vi "MultiChannnel_With_Origin_init_Matrix_FileIO.vi"() -> ()   [LabVIEW 2023]
uses:
  <vilib>/Waveform/WDTOps.llb/WDT Index Channel DBL.vi
  <vilib>/Analysis/NI_AALBase.lvlib
  <vilib>/Analysis/baseanly.llb/Mean (DBL).vi
  <vilib>/DAQmx/read.llb/DAQmx Read (Analog 1D Wfm NChan NSamp).vi
  <vilib>/Analysis/Matrix/NI_Matrix.lvlib
  <vilib>/Analysis/baseanly.llb/Real A x B.vi
  <vilib>/DAQmx/configure/timing.llb/DAQmx Timing (Sample Clock).vi
  <vilib>/DAQmx/create/channels.llb/DAQmx Create Channel (AI-Voltage-Basic).vi
  <vilib>/Analysis/Matrix/Numeric/Conversions/Matrix To Array - RM.vi
panel:
  out "attributes 2":variant
  out "attributes":variant
  out "Filename Out":path
  out "Data Writing":bool caption="Saving Data"
  in  "DataWriting SW":bool caption="Enable"
  out "Force Graph":dbl[][](graph)
  out "Force Array (F)   -> Time":dbl[][](array[numeric]) format="%#.3f"
  in  "Convert Matrix":dbl[][](array[numeric])=[[0.01787384, 0.5614992, -0.6825333], [-0.80829626, 0.31005788, 0.3553213], [0.6880116, 0.4358145, 0.7359737]]
  in  "StopAll":bool
  out "How many time get offset":i32
  out "Ch3 Origin":dbl
  out "Ch2 Origin":dbl
  out "Ch1 Origin":dbl
  out "RawCantilever (V)\n (Offset removed     -> Time)":dbl[][](array[numeric]) format="%#.3f"
  out "C 3":dbl[](array[numeric]) format="%#.5g"
  out "C 2":dbl[](array[numeric]) format="%#.5g"
  out "C1":dbl[](array[numeric]) format="%#.5g"
  in  "Get Orogin":bool
  out "Raw AD":waveform(dbl)[](graph)
  in  "samples per channel":i32=500
  in  "sample mode":i32(ring)=10123 items=["Continuous Samples"=10123, "Finite Samples"=10178, "Hardware Timed Single Point"=12522]
  in  "rate":dbl=1000.0 format="%0.2f"
  in  "physical channels":tag="Dev2/ai0:2"
  # "Phy Channel -> Set to 0-2\nRate 1000Hz\nSampleMode  -> Contenious Sampling\nSample per Channel -> 100"
  # "Raw A/D (V)"
  # "C1"
  # "Shear X"
  # "C2"
  # "Shear Y"
  # "Offset (V)"
  # "C3"
  # "Force Z"
  # "No.509 \n[[ 0.01787384, 0.5614992 , -0.6825333 ],\n[-0.80829626, 0.31005788, 0.3553213 ],\n[ 0.6880116 , 0.4358145 , 0.7359737 ]"
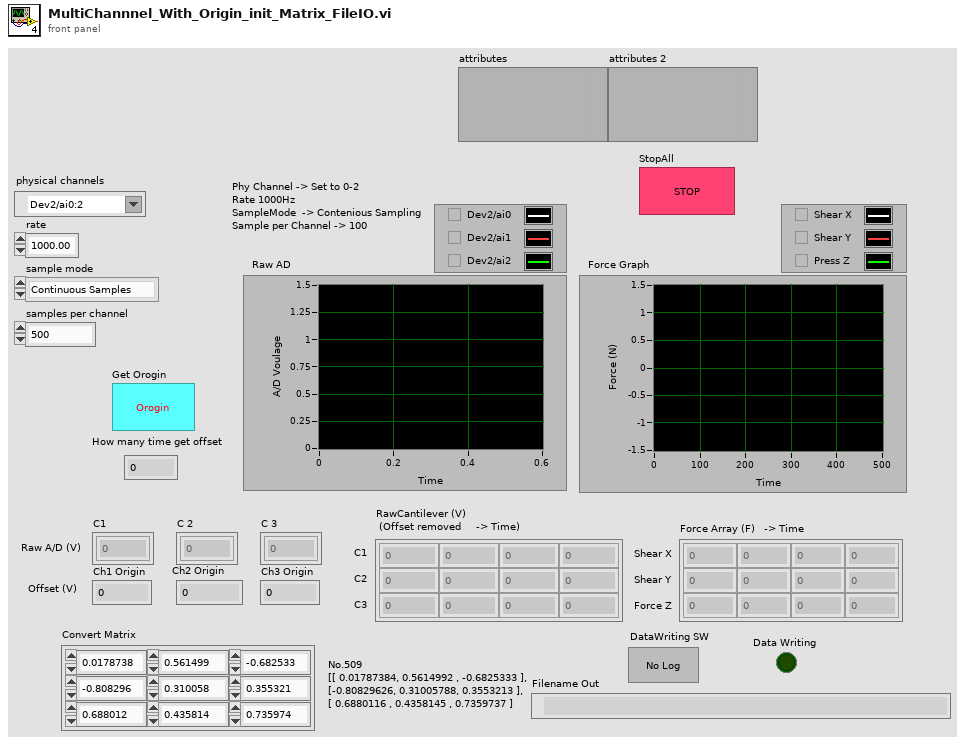
[diagram p1: front panel]
types:
  T1 = typedef "NI_Matrix.lvlib/RealMatrix.ctl" = dbl[][]
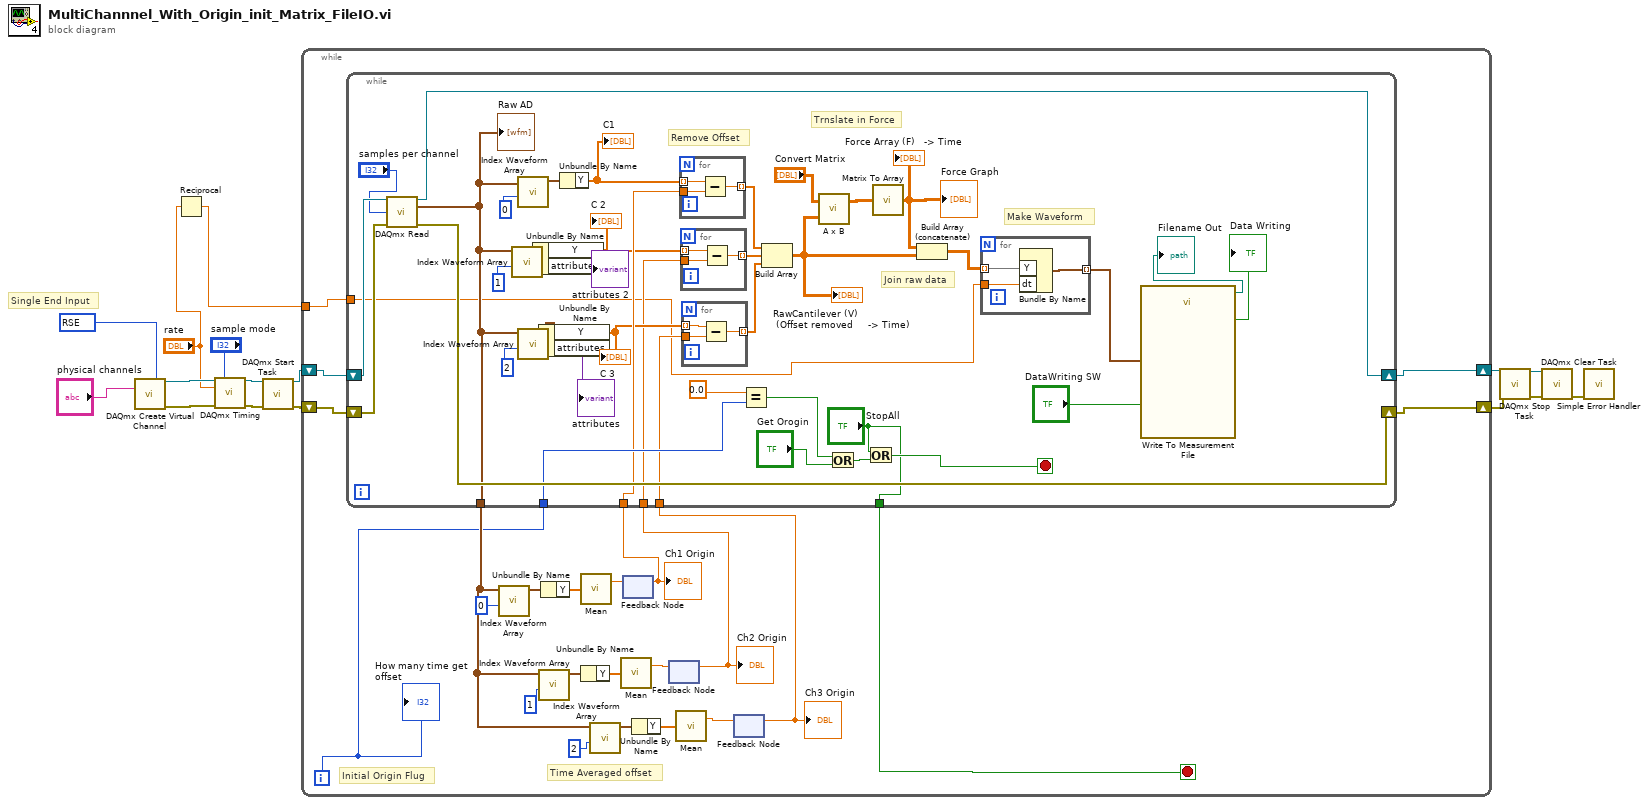
[diagram p0: block diagram]
diagram:
  w3 = 10083 items=["Default"=-1, "RSE"=10083, "NRSE"=10078, "Differential"=10106, "Pseudodifferential"=12529] ("input terminal configuration")
  # "Single End Input"
  n1 = call-poly <vilib>:"DAQmx Create Virtual Channel.vi"("input terminal configuration"=w3, "physical channels"="physical channels") -> ("task out"=w8:refnum<k21>, "error out"=w7:errorcluster)  [unwired: 12 in]
  n2 = Reciprocal(x="rate") -> (1/x=w1:dbl)
  n3 = call-poly <vilib>:"DAQmx Timing.vi"("task/channels in"=w8, "sample mode"="sample mode", "rate"="rate", "error in"=w7) -> ("task out"=w6:refnum<k21>, "error out"=w5:errorcluster)  [unwired: 10 in]
  n4 = call <vilib>:"DAQmx Start Task.vi"("task/channels in"=w6, "error in"=w5) -> ("task out"=w15:refnum<k21>, "error out"=w14:errorcluster)  [unwired: 12 in]
  n5 = while {
    shift-right: [w36] -> w12
    shift-left: w15 -> [w39]
    shift-right: [w37] -> w13
    shift-left: w14 -> [w38]
    tunnel: w1 -> [w17]
    i -> [w27]
    stop <- w28 stop-if-true
    # "Time Averaged offset"
    # "Initial Origin Flug"
    n6 = feedback #1() -> (w23:dbl)  [unwired: 1 in]
    "Ch1 Origin" <- w23
    n7 = feedback #2() -> (w18:dbl)  [unwired: 1 in]
    "Ch2 Origin" <- w18
    n8 = feedback #3() -> (w19:dbl)  [unwired: 1 in]
    "Ch3 Origin" <- w19
    n9 = while {
      shift-right: [w76] -> w36
      shift-left: w39 -> [w79]
      shift-right: [w77] -> w37
      shift-left: w38 -> [w78]
      tunnel: [w50] -> w32
      tunnel: ["StopAll"] -> w28
      tunnel: w27 -> [w65]
      tunnel: w23 -> [w58]
      tunnel: w18 -> [w54]
      tunnel: w19 -> [w53]
      tunnel: w17 -> [w47]
      stop <- w68 stop-if-true
      # "Make Waveform"
      # "Trnslate in Force"
      # "Remove Offset"
      # "Join raw data"
      n10 = call-poly <vilib>:"DAQmx Read.vi"("task/channels in"=w79, "number of samples per channel"="samples per channel", "error in"=w78) -> ("task out"=w76:refnum<k21>, "data"=w50:waveform(dbl)[], "error out"=w77:errorcluster)  [unwired: 10 in]
      "Raw AD" <- w50
      n11 = call-poly <vilib>:"Index Waveform Array.vi"("index"=1, "waveform array"=w50) -> ("waveform"=w71:waveform(dbl))  [unwired: 8 in, 1 out]
      n12 = call-poly <vilib>:"Index Waveform Array.vi"("index"=0, "waveform array"=w50) -> ("waveform"=w73:waveform(dbl))  [unwired: 8 in, 1 out]
      n13 = call-poly <vilib>:"Index Waveform Array.vi"("index"=2, "waveform array"=w50) -> ("waveform"=w69:waveform(dbl))  [unwired: 8 in, 1 out]
      n14 = Unbundle By Name(w71) -> ("Y"=w56:dbl[], "attributes"=→"attributes 2":variant)
      "C 2" <- w56
      n15 = Unbundle By Name(w69) -> ("Y"=w55:dbl[], "attributes"=→"attributes":variant)
      "C 3" <- w55
      n16 = Unbundle By Name(w73) -> ("Y"=w59:dbl[])
      "C1" <- w59
      n17 = for {
        tunnel: w59 -> [w91] mode=indexing
        tunnel: w58 -> [w90]
        tunnel: [w89] -> w57 mode=indexing
        n18 = Subtract(x=w91, y=w90) -> (x-y=w89:dbl)
      }
      n19 = for {
        tunnel: [w88] -> w52 mode=indexing
        tunnel: w56 -> [w87] mode=indexing
        tunnel: w54 -> [w86]
        n20 = Subtract(x=w87, y=w86) -> (x-y=w88:dbl)
      }
      n21 = for {
        tunnel: [w85] -> w51 mode=indexing
        tunnel: w55 -> [w84] mode=indexing
        tunnel: w53 -> [w83]
        n22 = Subtract(x=w84, y=w83) -> (x-y=w85:dbl)
      }
      n23 = Equal?(x=0.0, y=w65) -> (x = y?=w64:bool)
      n24 = Build Array(w57, w52, w51) -> (w45:dbl[][])
      "RawCantilever (V)\n (Offset removed     -> Time)" <- w45
      n25 = call-poly <vilib>:"A x B.vi"("B"=w45, "A"="Convert Matrix") -> ("A x B"=w61:T1)  [unwired: 1 out]
      n26 = Or(x=w64, y="Get Orogin") -> (x .or. y?=w62:bool)
      n27 = Or(x="StopAll", y=w62) -> (x .or. y?=w68:bool)
      n28 = call-poly <vilib>:"Matrix To Array.vi"("Real Matrix"=w61) -> ("Real 2D Array"=w43:dbl[][])
      "Force Array (F)   -> Time" <- w43
      "Force Graph" <- w43
      n29 = Build Array (concatenate)(w43, w45) -> (w44:dbl[][])
      n30 = for {
        tunnel: w44 -> [w80] mode=indexing
        tunnel: [w82] -> w46 mode=indexing
        tunnel: w47 -> [w81]
        n31 = Bundle By Name("Y"=w80, "dt"=w81) -> (w82:waveform(dbl))  [unwired: 1 in]
      }
      n32 = call "Write To Measurement File"("Signals"=w46, "Enable"="DataWriting SW") -> ("Filename Out"=→"Filename Out":path, "Saving Data"=→"Data Writing":bool)  [unwired: 15 in, 1 out]
    }
    n33 = call-poly <vilib>:"Index Waveform Array.vi"("index"=0, "waveform array"=w32) -> ("waveform"=w35:waveform(dbl))  [unwired: 8 in, 1 out]
    n34 = call-poly <vilib>:"Index Waveform Array.vi"("index"=1, "waveform array"=w32) -> ("waveform"=w34:waveform(dbl))  [unwired: 8 in, 1 out]
    n35 = Unbundle By Name(w35) -> ("Y"=w26:dbl[])
    n36 = call-poly <vilib>:"Mean.vi"("X"=w26) -> ("mean"=w24:dbl)  [unwired: 1 out]
    n37 = Unbundle By Name(w34) -> ("Y"=w25:dbl[])
    n38 = call-poly <vilib>:"Index Waveform Array.vi"("index"=2, "waveform array"=w32) -> ("waveform"=w33:waveform(dbl))  [unwired: 8 in, 1 out]
    n39 = call-poly <vilib>:"Mean.vi"("X"=w25) -> ("mean"=w22:dbl)  [unwired: 1 out]
    n40 = feedback-in #1(w24) -> ()
    n41 = Unbundle By Name(w33) -> ("Y"=w21:dbl[])
    n42 = feedback-in #2(w22) -> ()
    n43 = call-poly <vilib>:"Mean.vi"("X"=w21) -> ("mean"=w20:dbl)  [unwired: 1 out]
    n44 = feedback-in #3(w20) -> ()
    "How many time get offset" <- w27
  }
  n45 = call <vilib>:"DAQmx Stop Task.vi"("task/channels in"=w12, "error in"=w13) -> ("task out"=w10:refnum<k21>, "error out"=w11:errorcluster)  [unwired: 12 in]
  n46 = call <vilib>:"DAQmx Clear Task.vi"("task in"=w10, "error in"=w11) -> ("error out"=w9:errorcluster)  [unwired: 13 in]
  n47 = call <vilib>:"Simple Error Handler.vi"("error in (no error)"=w9) -> ()  [unwired: 4 in, 5 out]
